vi "TestLibGetStringArray.vi"() -> ()   [LabVIEW 2020]
uses:
  TestLabviewTools32.dll
panel:
  out "cFilePath":string
  out "fResult":i32
  out "Array":string[](array[string])
  in  "Path":path=path "C:/Factory/FactoryProductTestTool/FPTT_Setup.ini"
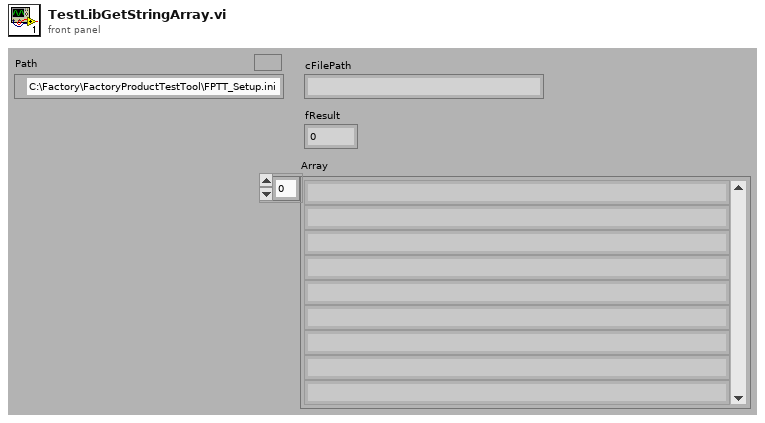
[diagram p1: front panel]
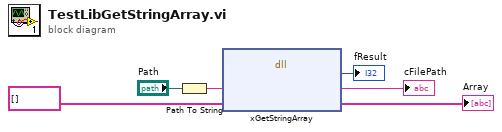
[diagram p0: block diagram]
diagram:
  n1 = Path To String(path="Path") -> (string=w1:string)
  n2 = dll-call lib="C:/Factory/FactoryGenericTools/Dll/TestLabviewTools32.dll" fn="xGetStringArray"("cFilePath"=w1, "vDataArray"=string[] [] ("Array")) -> ("fResult"=→"fResult":i32, "cFilePath"=→"cFilePath":string, "vDataArray"=→"Array":string[])  [unwired: 3 in, 2 out]
